vi "Send cmd S4ICS no delay.vi"(8 "error in (no error)":errorcluster, 10 "connection ID":refnum<k5>, 11 "data in":string) -> (0 "error out":errorcluster, 3 "data out":string)   [LabVIEW 2018]
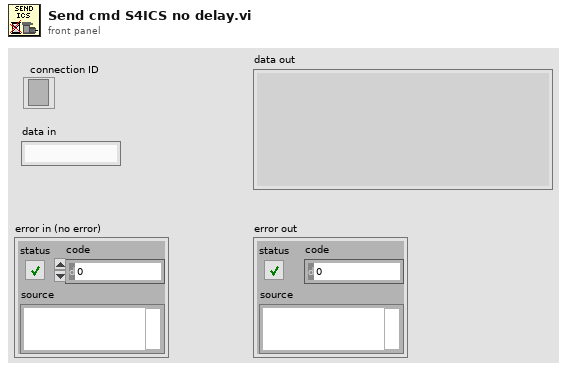
[diagram p1: front panel]
types:
  T1 = enum16{"Standard", "Buffered", "CRLF", "Immediate"}
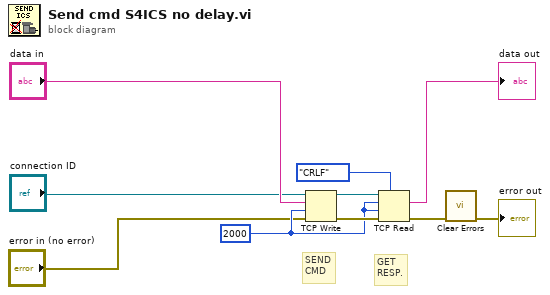
[diagram p0: block diagram]
diagram:
  w8 = 2000 ("bytes to read")
  # "GET\nRESP."
  # "SEND\nCMD"
  n1 = TCP Write(connection ID="connection ID", data in="data in", error in (no error)="error in (no error)", 9:w8) -> (connection ID out=w10:refnum<k5>, error out=w9:errorcluster)  [unwired: 1 out]
  n2 = TCP Read(connection ID=w10, bytes to read=w8, error in (no error)=w9, 7:T1."CRLF" ("mode (standard)"), 9:w8) -> (data out=→"data out":string, error out=w5:errorcluster)  [unwired: 1 out]
  n3 = call <vilib>:"Clear Errors.vi"("error in (no error)"=w5) -> ("error out"=→"error out":errorcluster)  [unwired: 5 in, 1 out]
